vi "AsyncEngine.vi"(8 "Error In":errorcluster, 10 "MicronGRPCClient in":refnum<class "MicronGRPCClient.lvclass">, 11 "AsyncDVR":refnum<data-value>) -> (0 "Error Out":errorcluster)   [LabVIEW 2019, in "MicronGRPCClient.lvclass"]
uses:
  MicronGRPCClient.lvclass
  Typedefs/AsyncCluster.ctl
  <vilib>/SLL Toolkit/SLL Queued State Machine/Queue Driver/Typedefs/Queue Type.ctl
  Typedefs/AsyncMessageRequest.ctl
  Generated/MicronGRPCGeneratedClient/RPC Messages/micronGrpc_MessageRequest.ctl
  Typedefs/AsyncMessageResponse.ctl
  <vilib>/Utility/error.llb/DialogType.ctl
  188d1d44-0cb4-4525-be29-801710e1132c.vi
  <vilib>/SLL Toolkit/SLL Queued State Machine/Queue Driver/Enqueue an Item to Queue.vi
  <vilib>/SLL Toolkit/SLL Queued State Machine/Queue Driver/Enqueue N Items.vi
  <vilib>/SLL Toolkit/SLL Queued State Machine/Queue Driver/Flush Queue.vi
  <vilib>/SLL Toolkit/SLL Queued State Machine/Queue Driver/Release Queue.vi
  <vilib>/SLL Toolkit/SLL Queued State Machine/SLL QSM.lvlib
  Generated/MicronGRPCGeneratedClient/MicronGRPCGeneratedClient.lvlib
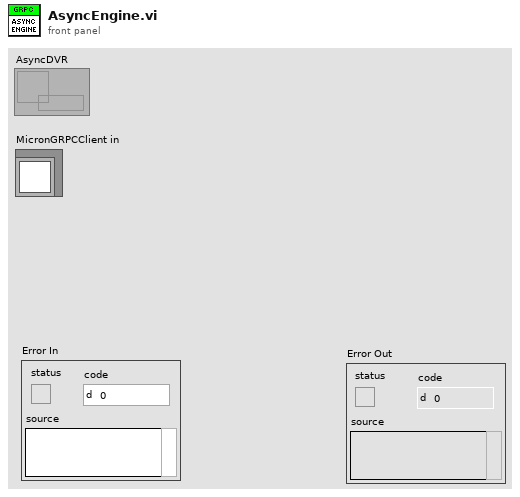
[diagram p1: front panel]
types:
  T1 = cluster{"Flags":cluster{"Source Code?":bool}, "AsyncDVR":refnum<data-value>}
  T2 = typedef "MicronGRPCClient.lvclass/AsyncCluster.ctl" = cluster{"InputQueue":refnum<queue>, "OutputQueue":refnum<queue>}
  T3 = typedef "MicronGRPCClient.lvclass/AsyncMessageResponse.ctl" = cluster{"Request":T4, "Collect Response?":bool, "Response":string, "error out":errorcluster}
  T4 = typedef "MicronGRPCGeneratedClient.lvlib/micronGrpc_MessageRequest.ctl" = cluster{"command":string, "payload":string}
  T5 = typedef "MicronGRPCClient.lvclass/AsyncMessageRequest.ctl" = cluster{"Message":T4, "Timeout (ms)":i32, "Collect Response?":bool}
  T6 = typedef "SLL QSM.lvlib/Queue Type.ctl" = cluster{"State":string, "Data":variant}
  T7 = typedef "DialogType.ctl" = u16
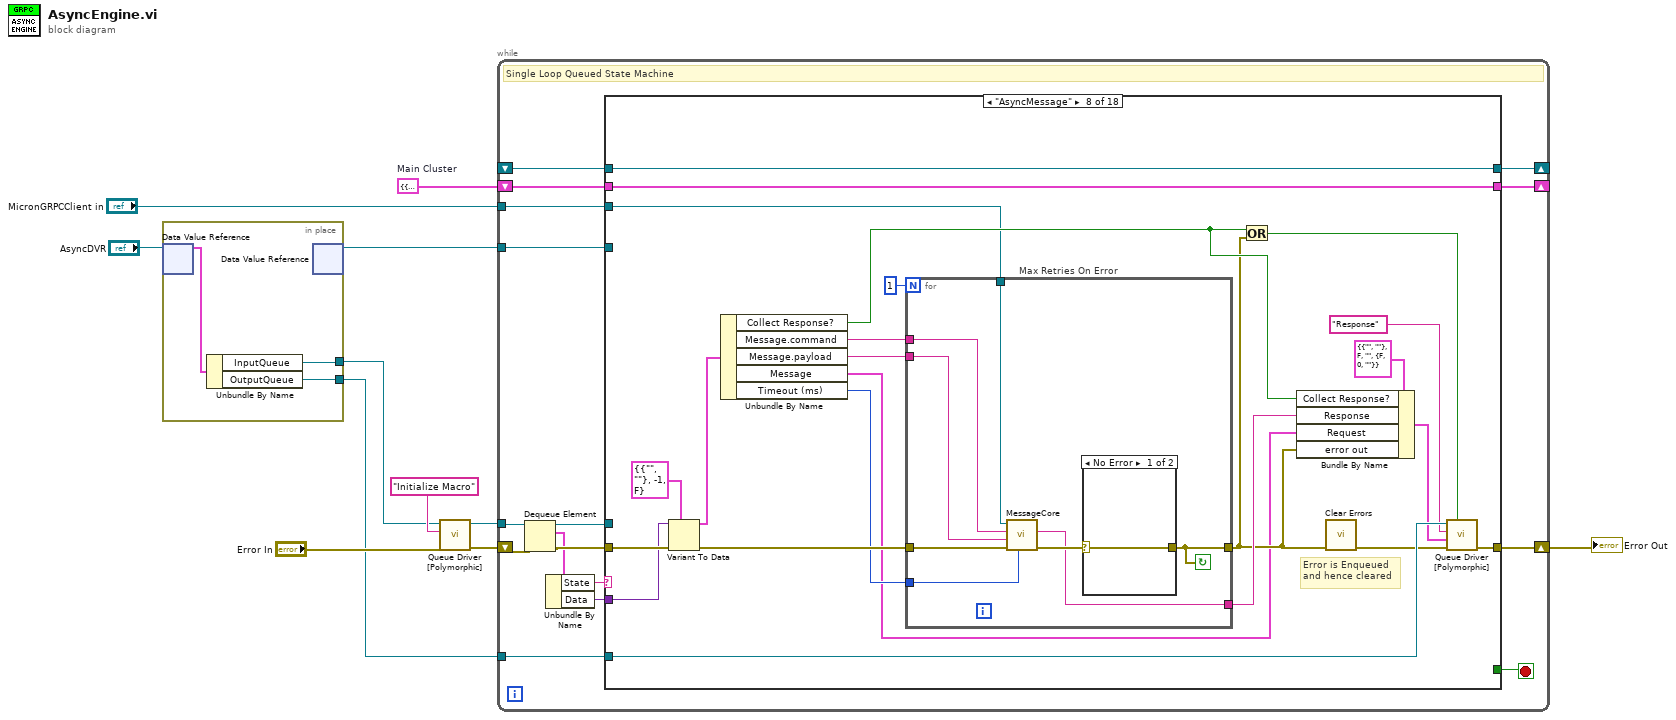
[diagram p0: block diagram]
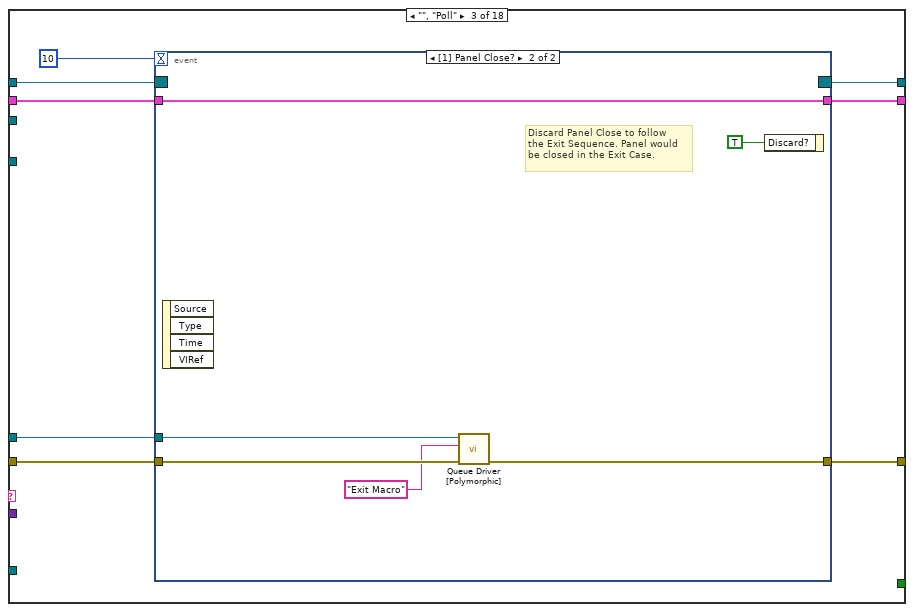
[diagram p4: hidden frame]
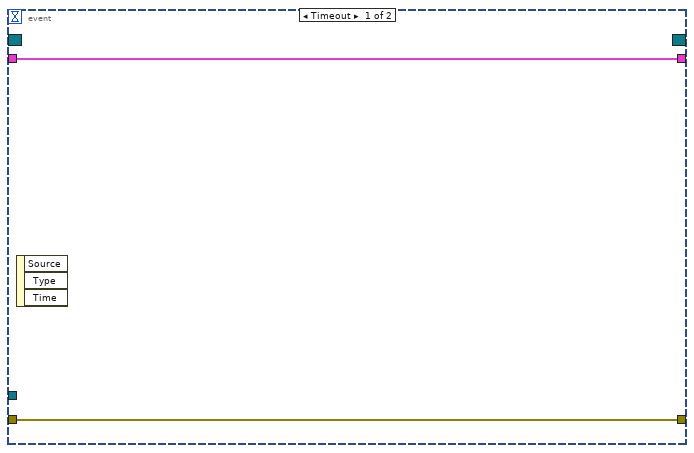
[diagram p5: hidden frame]
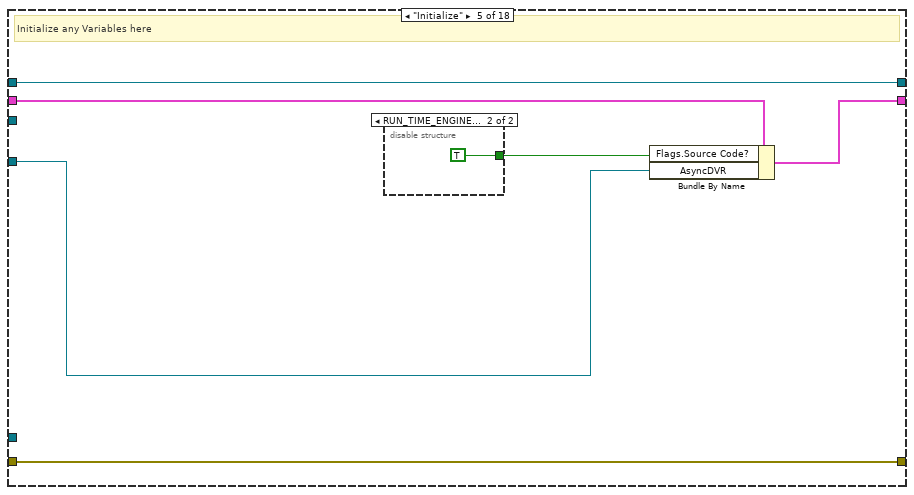
[diagram p7: hidden frame]
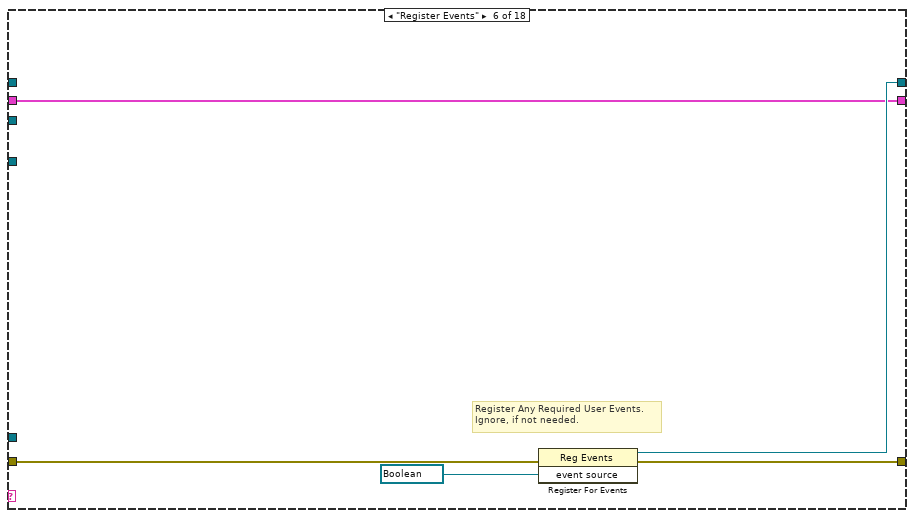
[diagram p9: hidden frame]
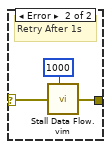
[diagram p11: hidden frame]
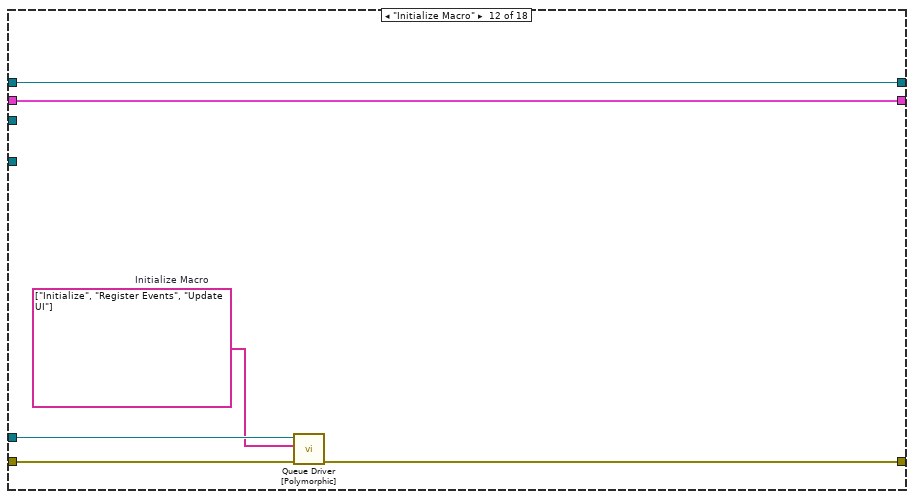
[diagram p15: hidden frame]
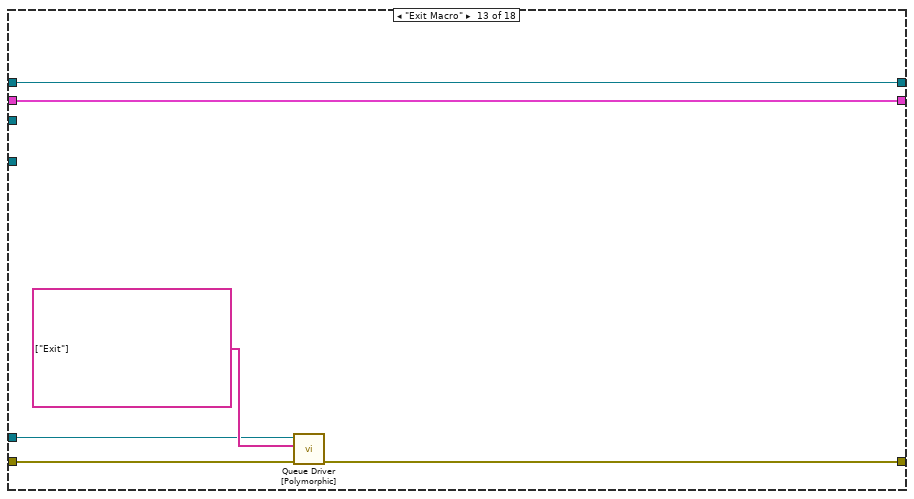
[diagram p16: hidden frame]
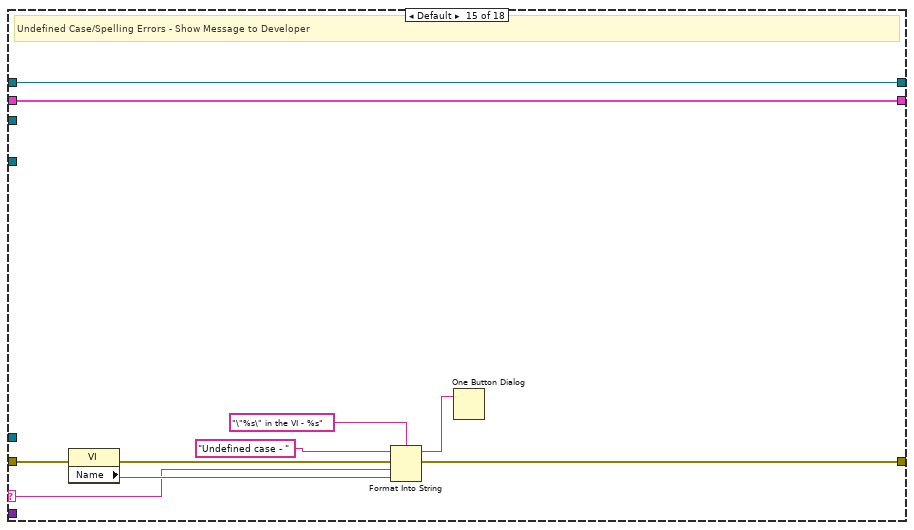
[diagram p18: hidden frame]
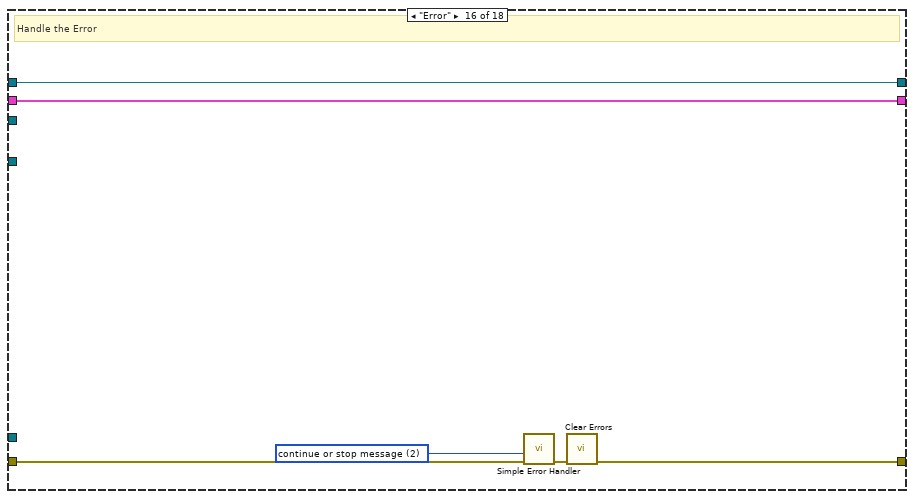
[diagram p19: hidden frame]
diagram:
  w9 = T1 {"Flags"={"Source Code?"=FALSE}, "AsyncDVR"=refnum}  # Main Cluster
  n1 = in-place {
    in-place-border: [w13] -> w4
    in-place-border: [w12] -> w2
    n2 = in-place-dvr #1("AsyncDVR") -> (w14:T2)  [unwired: 1 out]
    n3 = Unbundle By Name(w14) -> ("InputQueue"=w13:refnum<queue>, "OutputQueue"=w12:refnum<queue>)
    n4 = in-place-dvr #1() -> (w3:refnum<data-value>)  [unwired: 1 in, 1 out]
  }
  n5 = call-poly <vilib>:"Queue Driver [Polymorphic].vi"("Error In"="Error In", "Item to Add"="Initialize Macro", "Queue Ref In"=w4) -> ("Error Out"=w8:errorcluster, "Queue Ref Out"=w11:refnum<queue>)  [unwired: 7 in]
  n6 = while "SLL Queued State Machine" {
    shift-right: [w30] -> w6
    shift-left: w8 -> [w21]
    shift-right: [w28] -> _
    shift-left: _ -> [w27]
    shift-right: [w26] -> _
    shift-left: w9 -> [w25]
    tunnel: w11 -> [w20]
    tunnel: w3 -> [w24]
    tunnel: w2 -> [w23]
    tunnel: "MicronGRPCClient in" -> [w22]
    stop <- w29 stop-if-true
    # "Single Loop Queued State Machine"
    n7 = Dequeue Element(queue=w20, error in (no error)=w21) -> (queue out=w18:refnum<queue>, element=w17:T6, error out=w19:errorcluster)  [unwired: 1 in, 1 out]
    n8 = Unbundle By Name(w17) -> ("State"=w16:string, "Data"=w15:variant)
    n9 = case "QSM Case Structure" shown="\"AsyncMessage\"" w16 {
      selector: w16 -> [_ _ _ _ _ _ _ _ _ _ _ _ _ _ w130 _ _ _]
      tunnel: w19 -> [w33 w36 w42 w55 w61 w67 w70 w93 w108 w111 w114 w118 w124 w129 w133 w145 w148 w155]
      tunnel: [w33 w36 w43 w55 w61 w66 w70 w84 w108 w111 w114 w117 w123 w129 w136 w143 w148 w150] -> w30
      tunnel: [_ _ _ _ _ _ _ _ _ _ _ _ _ _ _ _ _ TRUE] -> w29
      tunnel: [w32 w35 w41 w54 w60 w65 w69 w92 w107 w110 w113 w120 w126 w128 w139 w142 w147 w149] -> w28
      tunnel: w27 -> [w32 w35 w40 w54 w60 _ w69 w92 w107 w110 w113 w120 w126 w128 w139 w142 w147 w149]
      tunnel: [w31 w34 w38 w53 w57 w64 w68 w91 w106 w109 w112 w119 w125 w127 w138 w141 w146 w154] -> w26
      tunnel: w25 -> [w31 w34 w39 w53 w58 w64 w68 w91 w106 w109 w112 w119 w125 w127 w138 w141 w146 w154]
      tunnel: w18 -> [_ _ w37 _ _ _ _ _ _ _ _ w116 w121 _ _ _ _ w153]
      tunnel: w15 -> [_ _ _ _ _ _ _ w90 _ _ _ _ _ _ _ _ _ _]
      tunnel: w24 -> [_ _ _ _ w56 _ _ _ _ _ _ _ _ _ _ _ _ _]
      tunnel: w23 -> [_ _ _ _ _ _ _ w83 _ _ _ _ _ _ _ _ _ _]
      tunnel: w22 -> [_ _ _ _ _ _ _ w71 _ _ _ _ _ _ _ _ _ _]
      frame "/--------------- Read Me -----------------/" {
        # "General Purpose Queue Based State Machine for Any Use Case (main application, module, pop up message etc)\n\nAdvantages:\n1. Lean Project Code Base (dependencies are in vilib).\n2. This template can be safely used in multiple parallel running modules without any issues.\n3. This template can also be safely used even in cases where the VI is configured to be a clone, where multiple \ninstances of the VI could be executing concurrently.\n\nHow to Use:\n1. Add necessary items to the Main Cluster.\n2. Use the Polymorphic Queue Driver for doing any queue operations. \n3. Add any required user events in the \"Register Events\" case. Ignore if not needed.\n4. Use \"Macros\" section for defining any list of state calls, which could be used in multiple places. \nEx: Initialize Macro, might be needed if we need to any reinitialization."
      }
      frame "/------------------ Poll -------------------/" {
      }
      frame "", "Poll" {
        n10 = event shown="[1] Panel Close?" {
          selector: w40 -> [_ _]
          dyn-events: [_ _] -> w41
          timeout: 10 -> [_ _]
          tunnel: [w46 w51] -> w43
          tunnel: w42 -> [w46 w52]
          tunnel: w39 -> [w45 w50]
          tunnel: [w45 w50] -> w38
          tunnel: w37 -> [_ w48]
          event Timeout {
            n11 = event-data() -> ()  [unwired: 1 in, 3 out]
          }
          event Panel Close? {
            # "Discard Panel Close to follow\nthe Exit Sequence. Panel would\nbe closed in the Exit Case."
            n12 = event-data() -> ()  [unwired: 1 in, 4 out]
            n13 = call-poly <vilib>:"Queue Driver [Polymorphic].vi"("Error In"=w52, "Item to Add"="Exit Macro" ("Enqueue"), "Queue Ref In"=w48) -> ("Error Out"=w51:errorcluster)  [unwired: 7 in, 1 out]
            n14 = event-data("Discard?"=TRUE) -> ()  [unwired: 1 in, 1 out]
          }
        }
      }
      frame "/--------------- Initialize -----------------/" {
      }
      frame "Initialize" {
        # "Initialize any Variables here"
        n15 = disable-structure shown="RUN_TIME_ENGINE==False" {
          disable-tunnel: [_ TRUE] -> w59
          frame condition #0 {
          }
          frame condition #1 (active) {
          }
        }
        n16 = Bundle By Name(cluster=w58, "Flags.Source Code?"=w59, "AsyncDVR"=w56) -> (w57:T1)
      }
      frame "Register Events" {
        # "Register Any Required User Events. \nIgnore, if not needed."
        n17 = register-events(error in=w67, refnum<vi> refnum ("event source")) -> (reference out=w65:refnum<event-registration>, error out=w66:errorcluster)  [unwired: 1 in]
      }
      frame "/---------- Custom Case Splitter ----------/" {
      }
      frame "AsyncMessage" {
        # "Error is Enqueued\nand hence cleared"
        n18 = Variant To Data(error in=w93, type=T5 {"Message"={"command"="", "payload"=""}, "Timeout (ms)"=-1, "Collect Response?"=FALSE} ("Async"), Variant=w90) -> (data=w87:T5, error out=w88:errorcluster)
        n19 = Unbundle By Name(w87) -> ("Collect Response?"=w79:bool, "Message.command"=w73:string, "Message.payload"=w72:string, "Message"=w74:T4, "Timeout (ms)"=w86:i32)
        n20 = for "Max Retries On Error" {
          N: 1 -> [_]
          tunnel: [w96] -> w78
          tunnel: w88 -> [w100]
          tunnel: [w101] -> w76
          tunnel: w86 -> [w97]
          tunnel: w71 -> [w98]
          tunnel: w73 -> [w95]
          tunnel: w72 -> [w94]
          stop <- w101 continue-if-true
          n21 = call-dynamic "MessageCore.vi"("Timeout (ms)"=w97, "error in (no error)"=w100, "Payload"=w94, "Command"=w95, "GRPCClient in"=w98) -> ("error out"=w99:errorcluster, "Response"=w96:string)  [unwired: 4 in, 1 out]
          n22 = case shown="No Error" w99 {
            selector: w99 -> [w102 w105]
            tunnel: [w102 w104] -> w101
            frame No Error {
            }
            frame Error {
              # "Retry After 1s"
              n23 = call "Stall Data Flow.vim"("value in"=w105, "milliseconds to wait"=u32 1000) -> ("value out"=w104:errorcluster)  [unwired: 1 out]
            }
          }
        }
        n24 = Or(x=w79, y=w76) -> (x .or. y?=w82:bool)
        n25 = Bundle By Name(cluster=T3 {"Request"={"command"="", "payload"=""}, "Collect Response?"=FALSE, "Response"="", "error out"={"status"=FALSE, "code"=0, "source"=""}} ("AsyncResponse"), "Collect Response?"=w79, "Response"=w78, "Request"=w74, "error out"=w76) -> (w80:T3)
        n26 = call <vilib>:"Clear Errors.vi"("error in (no error)"=w76) -> ("error out"=w75:errorcluster)  [unwired: 5 in, 1 out]
        n27 = call-poly <vilib>:"Queue Driver [Polymorphic].vi"("Add to Queue? (T)"=w82, "Error In"=w75, "Data (Optional)"=w80, "Item to Add"="Response", "Queue Ref In"=w83) -> ("Error Out"=w84:errorcluster)  [unwired: 5 in, 1 out]
      }
      frame "/-------------- User Interface --------------/" {
        # "Duplicate this case to create additional case splitters for readability"
      }
      frame "Update UI" {
        # "Update Front Panel Controls in this Case"
      }
      frame "/----------------- Macros -----------------/" {
      }
      frame "Initialize Macro" {
        w115 = string[] ["Initialize", "Register Events", "Update UI"]  # Initialize Macro
        n28 = call-poly <vilib>:"Queue Driver [Polymorphic].vi"("Error In"=w118, "Enqueue N"=w115, "Queue Ref In"=w116) -> ("Error Out"=w117:errorcluster)  [unwired: 7 in, 1 out]
      }
      frame "Exit Macro" {
        n29 = call-poly <vilib>:"Queue Driver [Polymorphic].vi"("Error In"=w124, "Enqueue N"=string[] ["Exit"], "Queue Ref In"=w121) -> ("Error Out"=w123:errorcluster)  [unwired: 7 in, 1 out]
      }
      frame "/-------------- Error Handler--------------/" {
      }
      frame Default {
        # "Undefined Case/Spelling Errors - Show Message to Developer"
        n30 = property class="VI"(error in=w133) -> (error out=w132:errorcluster, "Name"=w131:string)  [unwired: 1 in, 1 out]
        n31 = Format Into String(format string="\"%s\" in the VI - %s" ("message"), initial string="Undefined case - ", error in=w132, w130, w131) -> (resulting string=w134:string, error out=w136:errorcluster)
        n32 = One Button Dialog(message=w134) -> ()  [unwired: 1 in, 1 out]
      }
      frame "Error" {
        w140 = T7 2 items=["no dialog", "OK message", "continue or stop message", "OK message + warnings", "continue/stop + warnings"] ("type of dialog (OK msg:1)")
        # "Handle the Error"
        n33 = call <vilib>:"Simple Error Handler.vi"("type of dialog (OK msg:1)"=w140, "error in (no error)"=w145) -> ("error out"=w144:errorcluster)  [unwired: 3 in, 4 out]
        n34 = call <vilib>:"Clear Errors.vi"("error in (no error)"=w144) -> ("error out"=w143:errorcluster)  [unwired: 5 in, 1 out]
      }
      frame "/------------------- Exit --------------------/" {
      }
      frame "Exit" {
        n35 = call-poly <vilib>:"Queue Driver [Polymorphic].vi"("Error In"=w155, "Queue Ref In"=w153) -> ("Error Out"=w156:errorcluster, "Queue Ref Out"=w152:refnum<queue>)  [unwired: 7 in, 1 out]
        n36 = call-poly <vilib>:"Queue Driver [Polymorphic].vi"("Error In"=w156, "Queue Ref In"=w152) -> ("Error Out"=w151:errorcluster)  [unwired: 9 in]
        n37 = Unregister For Events(event registration refnum=w149, error in=w151) -> (error out=w150:errorcluster)
      }
    }
  }
  "Error Out" <- w6
